vi "pro.vi"() -> ()   [LabVIEW 2018]
uses:
  <vilib>/Utility/file.llb/Write Delimited Spreadsheet (string).vi
  <vilib>/Utility/file.llb/Write Delimited Spreadsheet (DBL).vi
panel:
  in  "Tab Control":T1(tab)
  out "?":dbl[][](graph)
  out "Umiditate":dbl(graph)
  out "Temperatura":dbl(graph)
  out "Presiune":dbl(graph)
  out "Elapsed Time (s)":dbl format="%#_2g"
  out "date/time string":string
  in  "Milisecunde to wait":u32(slide) scale=0.0..1000.0
  out "file or folder exists?":bool
  out "appended array":dbl[][](array[numeric])
  out "Array":string[](array[string])
  in  "stop":bool
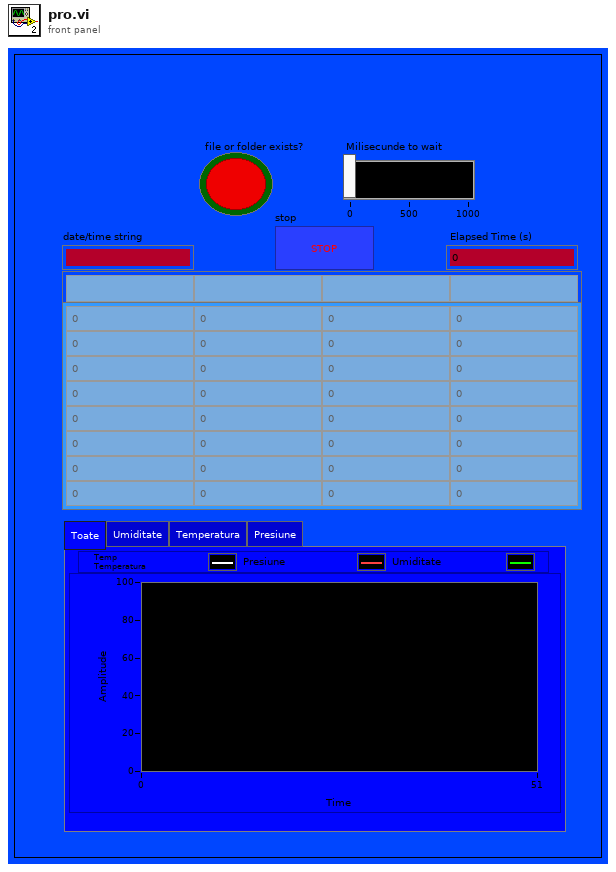
[diagram p1: front panel]
types:
  T1 = enum32{"Toate", "Umiditate", "Temperatura", "Presiune"}
  T2 = enum16{"open", "replace", "create", "open or create", "replace or create", "replace or create with confirmation"}
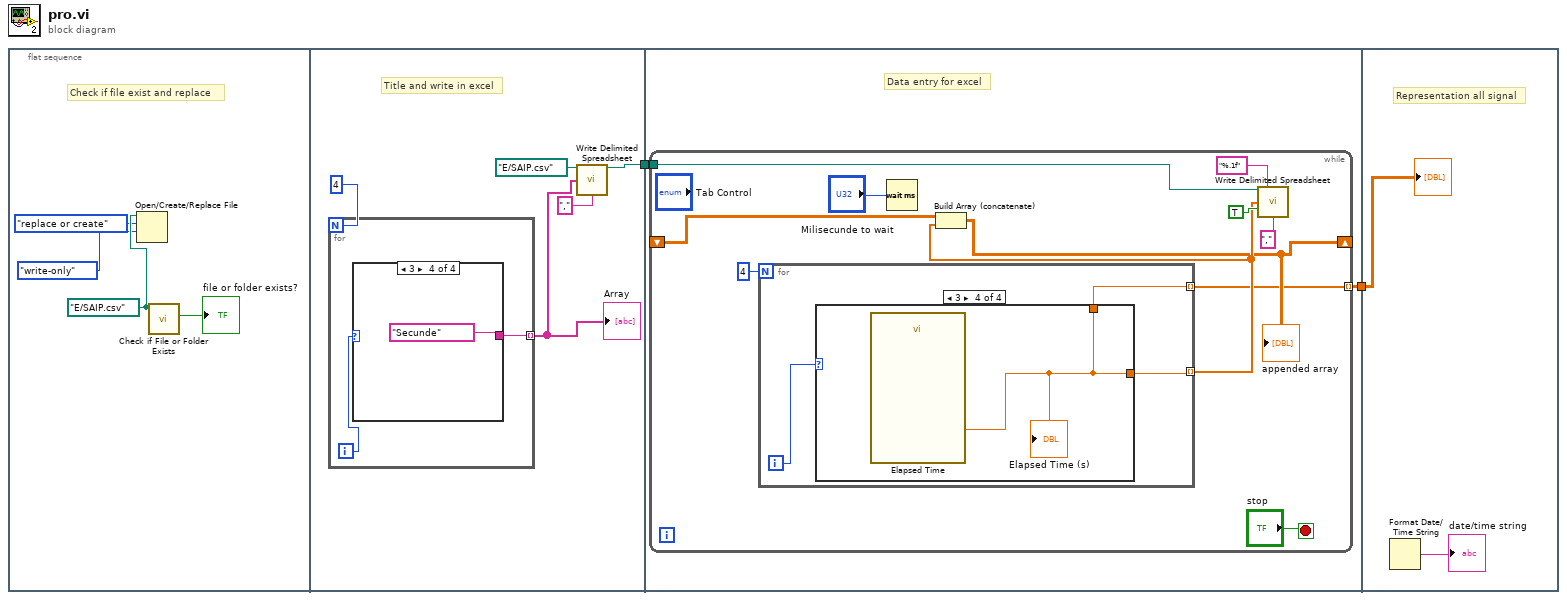
[diagram p0: block diagram]
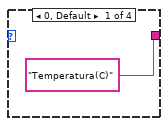
[diagram p2: hidden frame]
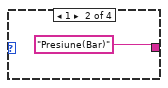
[diagram p3: hidden frame]
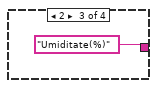
[diagram p4: hidden frame]
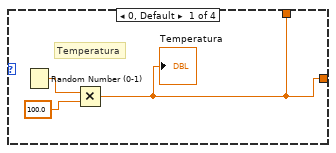
[diagram p5: hidden frame]
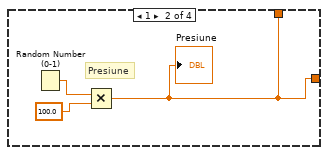
[diagram p6: hidden frame]
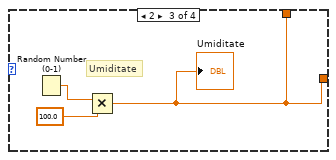
[diagram p7: hidden frame]
diagram:
  n1 = flat-sequence {
    tunnel: [w10] -> w2
    tunnel: w2 -> [w19]
    tunnel: [w18] -> w1
    tunnel: w1 -> [w45]
    frame #0 {
      w5 = path "E:/SAIP.csv" ("path")
      # "Check if file exist and replace"
      n2 = Open/Create/Replace File(file path (use dialog)=w5, operation (0:open)=T2."replace or create", access (0:read/write)=enum16{"read/write", "read-only", "write-only"}."write-only") -> ()  [unwired: 3 in, 3 out]
      n3 = call <vilib>:"Check if File or Folder Exists.vi"("path"=w5) -> ("file or folder exists?"=→"file or folder exists?":bool)  [unwired: 8 in, 2 out]
    }
    frame #1 {
      # "Title and write in excel"
      n4 = for {
        N: 4 -> [_]
        tunnel: [w12] -> w7 mode=indexing
        i -> [w13]
        n5 = case shown="3" w13 {
          tunnel: ["Temperatura(C)" "Presiune(Bar)" "Umiditate(%)" "Secunde"] -> w12
          frame 0, Default {
          }
          frame 1 {
          }
          frame 2 {
          }
          frame 3 {
          }
        }
      }
      "Array" <- w7
      n6 = call-poly <vilib>:"Write Delimited Spreadsheet.vi"("file path (dialog if empty)"=path "E:/SAIP.csv", "1D data"=w7, "delimiter (\\t)"="," ("delimiter (\\t)")) -> ("new file path (Not A Path if cancelled)"=w10:path)  [unwired: 11 in, 1 out]
    }
    frame #2 {
      # "Data entry for excel"
      n7 = while {
        tunnel: w19 -> [w28]
        shift-right: [w22] -> _
        shift-left: _ -> [w25]
        tunnel: [w21] -> w18 mode=indexing
        stop <- "stop" stop-if-true
        n8 = for {
          N: 4 -> [_]
          tunnel: [w31] -> w24 mode=indexing
          tunnel: [w32] -> w21 mode=indexing
          i -> [w33]
          n9 = case shown="3" w33 {
            tunnel: [w34 w37 w40 w43] -> w32
            tunnel: [w34 w37 w40 w43] -> w31
            frame 0, Default {
              # "Temperatura"
              n10 = Random Number (0-1)() -> (number: 0 to 1=w36:dbl)
              n11 = Multiply(x=w36, y=100.0) -> (x*y=w34:dbl)
              "Temperatura" <- w34
            }
            frame 1 {
              # "Presiune"
              n12 = Random Number (0-1)() -> (number: 0 to 1=w39:dbl)
              n13 = Multiply(x=w39, y=100.0) -> (x*y=w37:dbl)
              "Presiune" <- w37
            }
            frame 2 {
              # "Umiditate"
              n14 = Random Number (0-1)() -> (number: 0 to 1=w42:dbl)
              n15 = Multiply(x=w42, y=100.0) -> (x*y=w40:dbl)
              "Umiditate" <- w40
            }
            frame 3 {
              n16 = call "Elapsed Time"() -> ("Elapsed Time (s)"=w43:dbl)  [unwired: 12 in, 7 out]
              "Elapsed Time (s)" <- w43
            }
          }
        }
        n17 = Wait (ms)(milliseconds to wait="Milisecunde to wait") -> ()  [unwired: 1 out]
        n18 = Build Array (concatenate)(w25, w24) -> (w22:dbl[][])
        "appended array" <- w22
        n19 = call-poly <vilib>:"Write Delimited Spreadsheet.vi"("file path (dialog if empty)"=w28, "format (%.3f)"="%.1f", "1D data"=w24, "append to file? (new file:F)"=TRUE, "delimiter (\\t)"="," ("delimiter (\\t)")) -> ()  [unwired: 9 in, 2 out]
      }
    }
    frame #3 {
      # "Representation all signal"
      n20 = Format Date/Time String() -> (date/time string=→"date/time string":string)  [unwired: 3 in]
      "?" <- w45
    }
  }
